vi "Close session.vi"(8 "error in (no error)":errorcluster, 11 "Python Toolkit in":refnum<class "Python Toolkit.lvclass">) -> (0 "error out":errorcluster, 3 "Python Toolkit out":refnum<class "Python Toolkit.lvclass">)   [LabVIEW 2018, in "Python Toolkit.lvclass"]
doc: "Close python session"
uses:
  Python Toolkit.lvclass
  Python Toolkit.lvclass/Python Toolkit.ctl
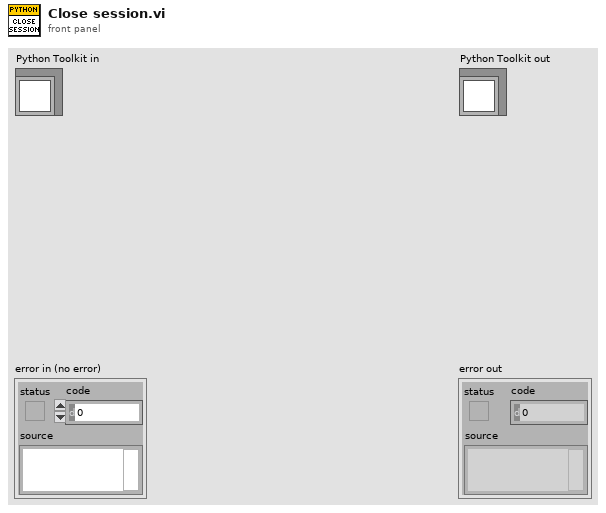
[diagram p1: front panel]
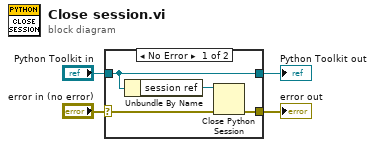
[diagram p0: block diagram]
diagram:
  n1 = case shown="No Error" "error in (no error)" {
    selector: "error in (no error)" -> [w7 w10]
    tunnel: [w6 w10] -> w3
    tunnel: [w8 w9] -> w1
    tunnel: "Python Toolkit in" -> [w8 w9]
    frame No Error {
      n2 = Unbundle By Name(w8) -> ("session ref"=w5:refnum<k35>)
      n3 = Close Python Session(session in=w5, error in=w7) -> (11:w6:errorcluster)
    }
    frame Error {
    }
  }
  "error out" <- w3
  "Python Toolkit out" <- w1
